vi "Scripting_FixControlTerminalLabel.vi"(8 "error in (no error)":errorcluster, 11 "ControlTerminalRef":refnum<vi>) -> (0 "error out":errorcluster, 3 "ChangedMade":bool)   [LabVIEW 2020]
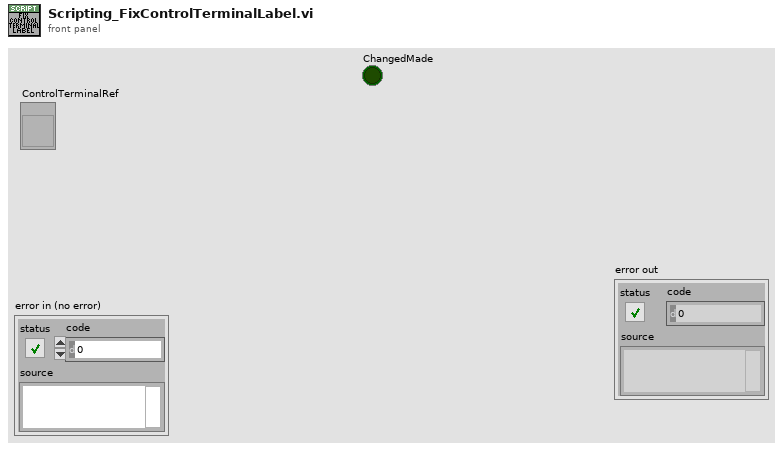
[diagram p1: front panel]
types:
  T1 = typedef "LVRectTypeDef.ctl" = cluster{"Left":i16, "Top":i16, "Right":i16, "Bottom":i16}
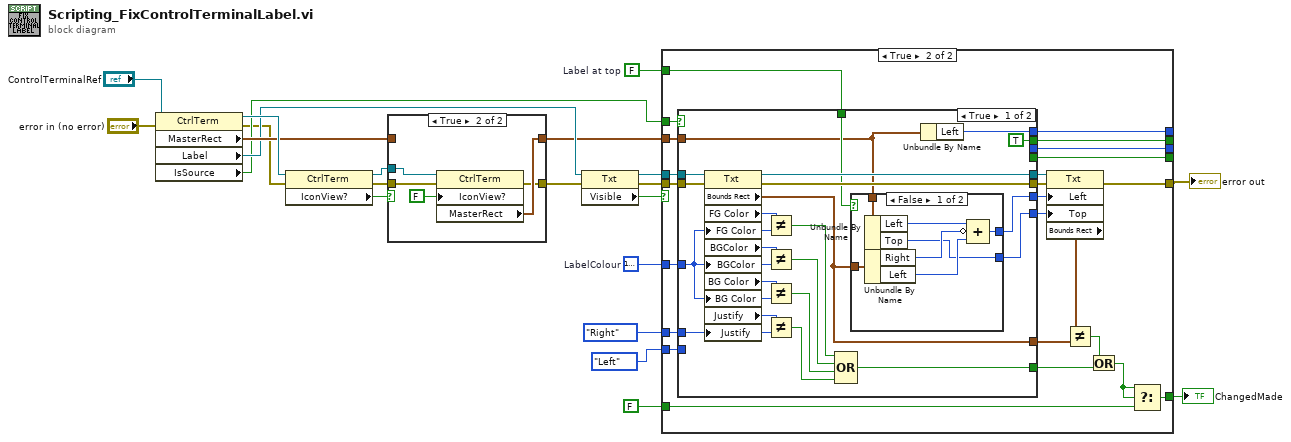
[diagram p0: block diagram]
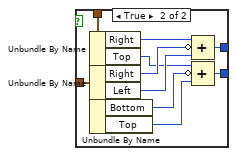
[diagram p3: hidden frame]
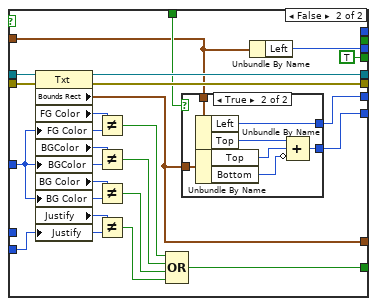
[diagram p4: hidden frame]
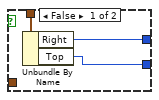
[diagram p5: hidden frame]
diagram:
  w9 = FALSE  # Label at top
  w8 = u32 16777216  # LabelColour
  n1 = property class="CtrlTerm"(reference="ControlTerminalRef", error in="error in (no error)") -> (reference out=w19:refnum<vi>, error out=w6:errorcluster, "MasterRect"=w18:T1, "Label"=w12:refnum<vi>, "IsSource"=w10:bool)
  n2 = property class="CtrlTerm"(reference=w19, error in=w6) -> (reference out=w22:refnum<vi>, error out=w21:errorcluster, "IconView?"=w20:bool)
  n3 = case shown="True" w20 {
    tunnel: w22 -> [_ w29]
    tunnel: w21 -> [w23 w28]
    tunnel: [w24 w26] -> w11
    tunnel: w18 -> [w24 _]
    tunnel: [w23 w25] -> w5
    frame False {
    }
    frame True {
      n4 = property class="CtrlTerm"(reference=w29, error in=w28, "IconView?"=FALSE ("Icon View?")) -> (error out=w25:errorcluster, "MasterRect"=w26:T1)  [unwired: 1 out]
    }
  }
  n5 = property class="Txt"(reference=w12, error in=w5) -> (reference out=w13:refnum<vi>, error out=w15:errorcluster, "Visible"=w14:bool)
  n6 = case shown="True" w14 {
    tunnel: w15 -> [w31 w55]
    tunnel: w11 -> [_ w54]
    tunnel: [w31 w33] -> w2
    tunnel: [w30 w34] -> w4
    tunnel: FALSE -> [w30 w35]
    tunnel: w8 -> [_ w53]
    tunnel: enum16{"Left", "Center", "Right"}."Right" ("Label.Justification") -> [_ w52]
    tunnel: enum16{"Left", "Center", "Right"}."Left" ("Label.Justification") -> [_ w51]
    tunnel: [_ w50] -> _
    tunnel: [_ w49] -> _
    tunnel: [_ w48] -> _
    tunnel: [_ w47] -> _
    tunnel: w13 -> [_ w46]
    tunnel: w10 -> [_ w45]
    tunnel: w9 -> [_ w32]
    frame False {
      # "Ignore Objects whose labels are not visible"
    }
    frame True {
      n7 = case shown="True" w45 {
        tunnel: w55 -> [w77 w115]
        tunnel: w54 -> [w56 w97]
        tunnel: [w63 w116] -> w40
        tunnel: w53 -> [w70 w109]
        tunnel: w52 -> [w68 _]
        tunnel: w51 -> [_ w107]
        tunnel: [w58 _] -> w50
        tunnel: [TRUE _] -> w49
        tunnel: [_ w96] -> w48
        tunnel: [_ TRUE] -> w47
        tunnel: w46 -> [w65 w103]
        tunnel: [w64 w101] -> w41
        tunnel: [w62 w95] -> w39
        tunnel: [w61 w100] -> w38
        tunnel: [w60 w99] -> w37
        tunnel: [w59 w102] -> w36
        tunnel: w32 -> [w57 w98]
        frame True {
          n8 = property class="Txt"(reference=w65, error in=w77, "FG Color"=w70, "BGColor"=w70, "BG Color"=w70, "Justify"=w68) -> (reference out=w64:refnum<vi>, error out=w63:errorcluster, "Bounds Rect"=w60:T1, "FG Color"=w76:u32, "BGColor"=w72:u32, "BG Color"=w71:u32, "Justify"=w69:enum16{"Left", "Center", "Right"})
          n9 = Not Equal?(x=w76, y=w70) -> (x != y?=w74:bool)
          n10 = Not Equal?(x=w72, y=w70) -> (x != y?=w75:bool)
          n11 = Not Equal?(x=w71, y=w70) -> (x != y?=w73:bool)
          n12 = Not Equal?(x=w69, y=w68) -> (x != y?=w67:bool)
          n13 = Compound Arithmetic op=OR(w74, w75, w73, w67) -> (w59:bool)
          n14 = case shown="False" w57 {
            tunnel: [w79 w88] -> w62
            tunnel: [w78 w87] -> w61
            tunnel: w60 -> [w84 w86]
            tunnel: w56 -> [w83 w85]
            frame False {
              n15 = Unbundle By Name(w83) -> ("Left"=w82:i16, "Top"=w78:i16)
              n16 = Unbundle By Name(w84) -> ("Right"=w81:i16, "Left"=w80:i16)
              n17 = Compound Arithmetic op=ADD(w82, invert w81, w80) -> (w79:i16)
            }
            frame True {
              n18 = Unbundle By Name(w85) -> ("Right"=w90:i16, "Top"=w89:i16)
              n19 = Unbundle By Name(w86) -> ("Right"=w94:i16, "Left"=w93:i16)
              n20 = Unbundle By Name(w86) -> ("Bottom"=w92:i16, "Top"=w91:i16)
              n21 = Compound Arithmetic op=ADD(w90, invert w94, w93) -> (w88:i16)
              n22 = Compound Arithmetic op=ADD(w89, invert w92, w91) -> (w87:i16)
            }
          }
          n23 = Unbundle By Name(w56) -> ("Left"=w58:i16)
        }
        frame False {
          n24 = property class="Txt"(reference=w103, error in=w115, "FG Color"=w109, "BGColor"=w109, "BG Color"=w109, "Justify"=w107) -> (reference out=w101:refnum<vi>, error out=w116:errorcluster, "Bounds Rect"=w99:T1, "FG Color"=w114:u32, "BGColor"=w110:u32, "BG Color"=w113:u32, "Justify"=w106:enum16{"Left", "Center", "Right"})
          n25 = Not Equal?(x=w114, y=w109) -> (x != y?=w112:bool)
          n26 = Not Equal?(x=w110, y=w109) -> (x != y?=w108:bool)
          n27 = Not Equal?(x=w113, y=w109) -> (x != y?=w111:bool)
          n28 = Not Equal?(x=w106, y=w107) -> (x != y?=w105:bool)
          n29 = Compound Arithmetic op=OR(w112, w108, w111, w105) -> (w102:bool)
          n30 = case shown="True" w98 {
            tunnel: w97 -> [w119 w123]
            tunnel: [w117 w122] -> w100
            tunnel: w99 -> [_ w121]
            tunnel: [w118 w120] -> w95
            frame False {
              n31 = Unbundle By Name(w119) -> ("Right"=w118:i16, "Top"=w117:i16)
            }
            frame True {
              n32 = Unbundle By Name(w123) -> ("Left"=w120:i16, "Top"=w126:i16)
              n33 = Unbundle By Name(w121) -> ("Top"=w125:i16, "Bottom"=w124:i16)
              n34 = Compound Arithmetic op=ADD(w126, w125, invert w124) -> (w122:i16)
            }
          }
          n35 = Unbundle By Name(w97) -> ("Left"=w96:i16)
        }
      }
      n36 = property class="Txt"(reference=w41, error in=w40, "Left"=w39, "Top"=w38) -> (error out=w33:errorcluster, "Bounds Rect"=w44:T1)  [unwired: 1 out]
      n37 = Not Equal?(x=w44, y=w37) -> (x != y?=w43:bool)
      n38 = Or(x=w43, y=w36) -> (x .or. y?=w42:bool)
      n39 = Select(t=w42, s=w42, f=w35) -> (s? t:f=w34:bool)
    }
  }
  "ChangedMade" <- w4
  "error out" <- w2
